vi "Actor1_GUI_G4_4.0.0_Create.vi"(8 "error in (no error)":errorcluster, 10 "LoopEvent":refnum<user-event>, 11 "reference in":refnum<class "Actor1_GUI_G4_4.0.0.lvclass">) -> (0 "error out":errorcluster, 3 "reference out":refnum<class "Actor1_GUI_G4_4.0.0.lvclass">)   [LabVIEW 2016, in "Actor1_GUI_G4_4.0.0.lvlib" / "Actor1_GUI_G4_4.0.0.lvclass"]
uses:
  <resource>/Framework/Providers/Open_GDS/ClassProviders/ActorFramework/4.0.0/Actor1_GUI_G4_4.0.0/Actor1_GUI_G4_4.0.0_Actor/Actor1_GUI_G4_4.0.0.lvclass
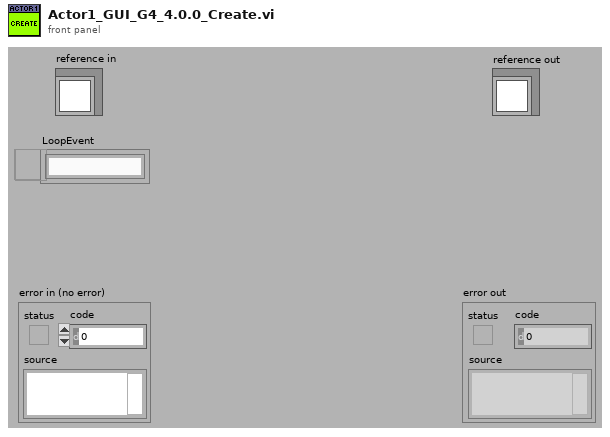
[diagram p1: front panel]
types:
  T1 = typedef "Actor1_GUI_G4_4.0.0.lvlib/Actor1_GUI_G4_4.0.0.lvclass/ObjectAttributes.ctl" = cluster{"LoopEvent":refnum<user-event>}
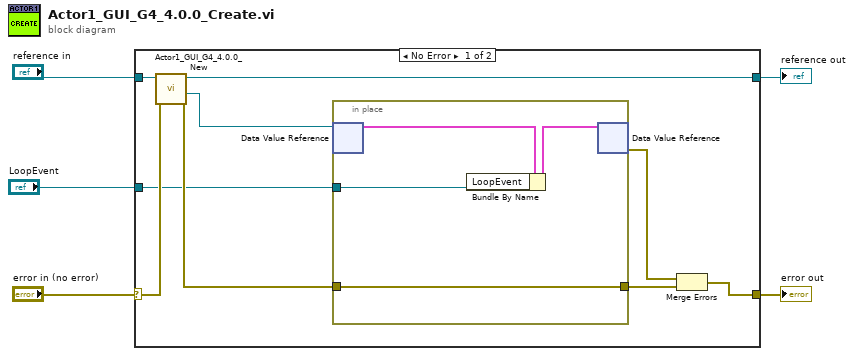
[diagram p0: block diagram]
diagram:
  n1 = case shown="No Error" "error in (no error)" {
    selector: "error in (no error)" -> [w13 w20]
    tunnel: [w10 w20] -> w4
    tunnel: "reference in" -> [w14 w19]
    tunnel: [w12 w19] -> w2
    tunnel: "LoopEvent" -> [w6 _]
    frame No Error {
      n2 = call <resource>:"Actor1_GUI_G4_4.0.0_New.vi"("error in (no error)"=w13, "reference in"=w14) -> ("error out"=w8:errorcluster, "DVRRefOut"=w9:refnum<data-value>, "reference out"=w12:refnum<class "Actor1_GUI_G4_4.0.0.lvclass">)  [unwired: 6 in, 1 out]
      n3 = in-place {
        in-place-border: w8 -> [w16]
        in-place-border: [w16] -> w7
        in-place-border: w6 -> [w15]
        n4 = in-place-dvr #1(w9) -> (w17:T1)  [unwired: 1 out]
        n5 = Bundle By Name(cluster=w17, "LoopEvent"=w15) -> (w18:T1)
        n6 = in-place-dvr #1(w18) -> (w11:errorcluster)  [unwired: 1 out]
      }
      n7 = Merge Errors(w11, w7) -> (w10:errorcluster)
    }
    frame Error {
    }
  }
  "error out" <- w4
  "reference out" <- w2
